vi "NI VeriStand - Save Model State.vi"(8 "error in (no error)":errorcluster, 10 "FilePath":path, 11 "Model in":T1) -> (0 "error out":errorcluster, 3 "Model out":T1)   [LabVIEW 2020, in "NI_VS Model ExecutionAPI.lvlib"]
doc: "Saves data about the current state of a model running on the target to a file you specify. You only can use this VI on your models and your compiled models you have built using The MathWorks, Inc. Simulink(R) software."
uses:
  <vilib>/NI VeriStand/Execution/Model/NI_VS Model ExecutionAPI.lvlib
  <vilib>/NI VeriStand/Execution/Model/ModelAPI.ctl
  NationalInstruments.VeriStand.ClientAPI
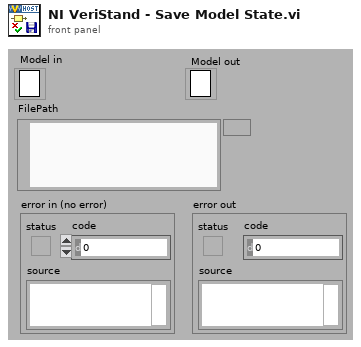
[diagram p1: front panel]
types:
  T1 = typedef "NI_VS Model ExecutionAPI.lvlib/ModelAPI.ctl" = refnum<k24>
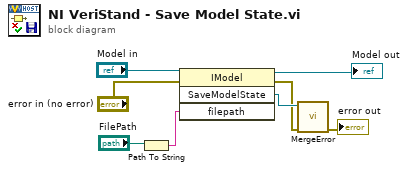
[diagram p0: block diagram]
diagram:
  n1 = Path To String(path="FilePath") -> (string=w1:string)
  n2 = invoke class="IModel" method="SaveModelState"(reference="Model in", error in="error in (no error)", "filepath"=w1) -> (reference out=→"Model out":T1, error out=w4:errorcluster, "SaveModelState"=w5:refnum<k24>)  [unwired: 1 in, 1 out]
  n3 = call <vilib>:"MergeError.vi"("error in (no error)"=w4, "Error"=w5) -> ("error out"=→"error out":errorcluster)  [unwired: 9 out]
